vi "Initialize Panel.vi"(8 "error in":errorcluster, 9 "MHL Configuration":T5, 10 "MHL References":T4, 11 "MHL UI Data in":T1) -> (0 "error out":errorcluster, 2 "MHL Data out":T3, 3 "MHL UI Data out":T1)   [LabVIEW 2017]
uses:
  controls/MHL References.ctl
  controls/MHL Configuration.ctl
  controls/MHL UI Data.ctl
  controls/MHL Status.ctl
  controls/MHL Data.ctl
  Boiler System Globals.vi
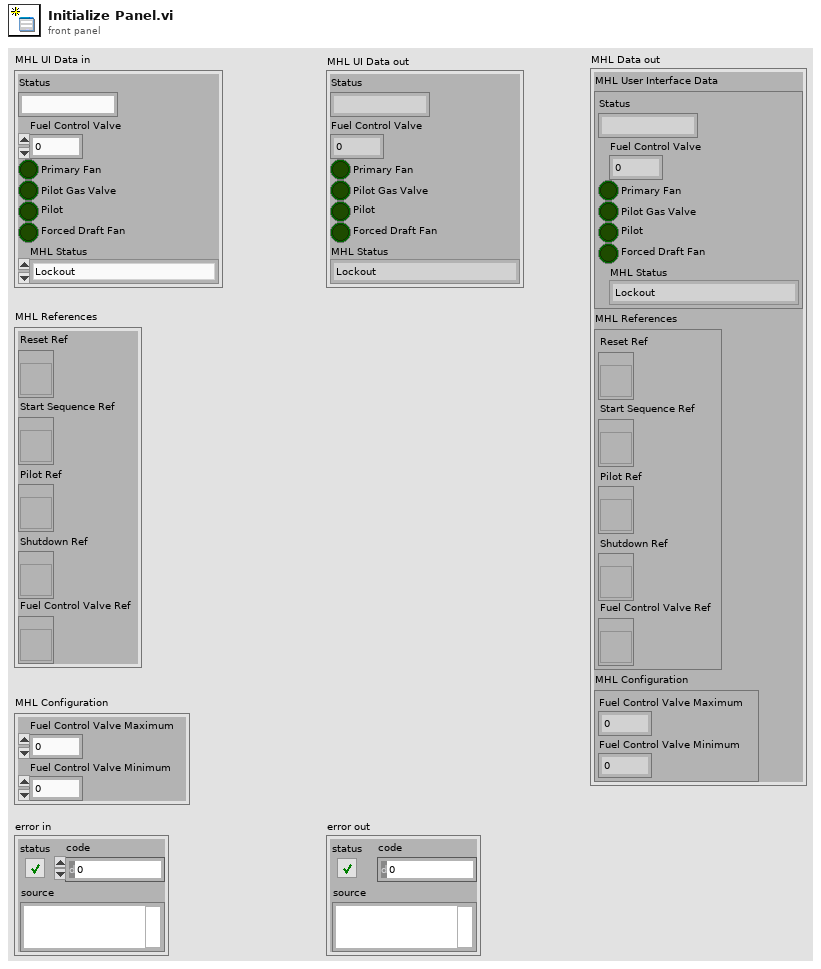
[diagram p1: front panel]
types:
  T1 = typedef "MHL UI Data.ctl" = cluster{"Status":string, "Fuel Control Valve":u32, "Primary Fan":bool, "Pilot Gas Valve":bool, "Pilot":bool, "Forced Draft Fan":bool, "MHL Status":T2}
  T2 = typedef "MHL Status.ctl" = enum16{"Lockout", "Ready", "Pre-Purge", "Pre-Purge Complete", "Pilot On", "Boiler Running", "Shutdown", "Purge"}
  T3 = typedef "MHL Data.ctl" = cluster{"MHL User Interface Data":T1, "MHL References":T4, "MHL Configuration":T5}
  T4 = typedef "MHL References.ctl" = cluster{"Reset Ref":refnum<vi>, "Start Sequence Ref":refnum<vi>, "Pilot Ref":refnum<vi>, "Shutdown Ref":refnum<vi>, "Fuel Control Valve Ref":refnum<vi>}
  T5 = typedef "MHL Configuration.ctl" = cluster{"Fuel Control Valve Maximum":dbl, "Fuel Control Valve Minimum":dbl}
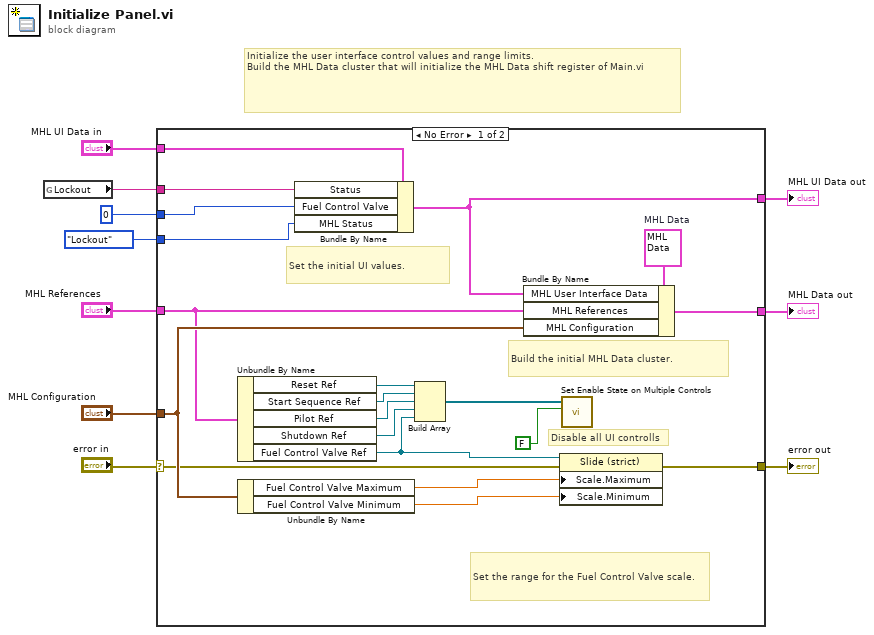
[diagram p0: block diagram]
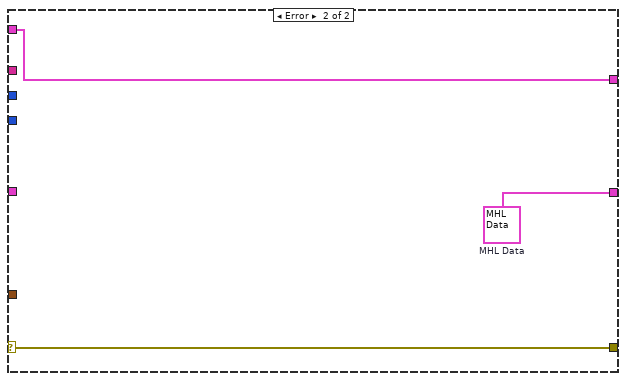
[diagram p2: hidden frame]
diagram:
  # "Initialize the user interface control values and range limits.\nBuild the MHL Data cluster that will initialize the MHL Data shift register of Main.vi"
  n1 = global read "Boiler System Globals.vi" "Lockout"() -> (w9:string)
  n2 = case shown="No Error" "error in" {
    selector: "error in" -> [w20 w33]
    tunnel: u32 0 ("Fuel Control Valve") -> [w28 _]
    tunnel: w9 -> [w27 _]
    tunnel: "MHL Configuration" -> [w25 _]
    tunnel: "MHL References" -> [w24 _]
    tunnel: "MHL UI Data in" -> [w23 w31]
    tunnel: [w22 w32] -> w5
    tunnel: [w21 w33] -> w4
    tunnel: [w19 w31] -> w2
    tunnel: MHL_Status."Lockout" ("MHL Status") -> [w18 _]
    frame No Error {
      w26 = T3 {"MHL User Interface Data"={"Status"="", "Fuel Control Valve"=0, "Primary Fan"=FALSE, "Pilot Gas Valve"=FALSE, "Pilot"=FALSE, "Forced Draft Fan"=FALSE, "MHL Status"=enum."Lockout"}, "MHL References"={"Reset Ref"=refnum, "Start Sequence Ref"=refnum, "Pilot Ref"=refnum, "Shutdown Ref"=refnum, "Fuel Control Valve Ref"=refnum}, "MHL Configuration"={"Fuel Control Valve Maximum"=0.0, "Fuel Control Valve Minimum"=0.0}}  # MHL Data
      # "Disable all UI controlls"
      # "Build the initial MHL Data cluster."
      # "Set the range for the Fuel Control Valve scale."
      # "Set the initial UI values."
      n3 = Unbundle By Name(w24) -> ("Reset Ref"=w17:refnum<vi>, "Start Sequence Ref"=w16:refnum<vi>, "Pilot Ref"=w15:refnum<vi>, "Shutdown Ref"=w14:refnum<vi>, "Fuel Control Valve Ref"=w13:refnum<vi>)
      n4 = Unbundle By Name(w25) -> ("Fuel Control Valve Maximum"=w30:dbl, "Fuel Control Valve Minimum"=w29:dbl)
      n5 = Bundle By Name(cluster=w23, "Status"=w27, "Fuel Control Valve"=w28, "MHL Status"=w18) -> (w19:T1)
      n6 = Build Array(w17, w16, w15, w14, w13) -> (w11:refnum<vi>[])
      n7 = Bundle By Name(cluster=w26, "MHL User Interface Data"=w19, "MHL References"=w24, "MHL Configuration"=w25) -> (w22:T3)
      n8 = property class="Slide (strict)"(reference=w13, error in=w20, "Scale.Maximum"=w30, "Scale.Minimum"=w29) -> (error out=w21:errorcluster)  [unwired: 1 out]
      n9 = call "Set Enable State on Multiple Controls.vi"("Enable?"=FALSE, "Controls"=w11) -> ()  [unwired: 10 in]
    }
    frame Error {
      w32 = T3 {"MHL User Interface Data"={"Status"="", "Fuel Control Valve"=0, "Primary Fan"=FALSE, "Pilot Gas Valve"=FALSE, "Pilot"=FALSE, "Forced Draft Fan"=FALSE, "MHL Status"=enum."Lockout"}, "MHL References"={"Reset Ref"=refnum, "Start Sequence Ref"=refnum, "Pilot Ref"=refnum, "Shutdown Ref"=refnum, "Fuel Control Valve Ref"=refnum}, "MHL Configuration"={"Fuel Control Valve Maximum"=0.0, "Fuel Control Valve Minimum"=0.0}}  # MHL Data
    }
  }
  "MHL Data out" <- w5
  "error out" <- w4
  "MHL UI Data out" <- w2
